vi "scale_waveform.vi"(2 "error in":errorcluster, 3 "waveform in":waveform(dbl)) -> (0 "error out":errorcluster, 1 "scaled waveform":waveform(dbl))   [LabVIEW 2017]
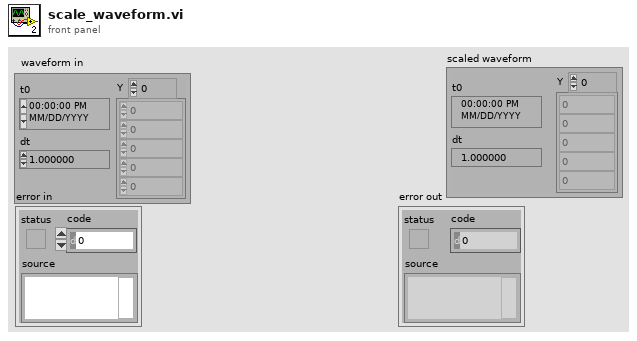
[diagram p1: front panel]
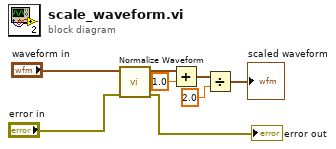
[diagram p0: block diagram]
diagram:
  n1 = call <vilib>:"Normalize Waveform.vi"("error in (no error)"="error in", "waveform in"="waveform in") -> ("error out"=→"error out":errorcluster, "normalized waveform"=w8:waveform(dbl))  [unwired: 6 in, 2 out]
  n2 = Add(x=w8, y=1.0) -> (x+y=w6:waveform(dbl))
  n3 = Divide(x=w6, y=2.0) -> (x/y=→"scaled waveform":waveform(dbl))
